vi "Get Tables.vi"(8 "error in (no error)":errorcluster, 11 "xwpfDocument in":refnum<class "xwpfDocument.lvclass">) -> (0 "error out":errorcluster, 2 "Tables":refnum<class "xwpfTable.lvclass">[](array[class]), 3 "xwpfDocument out":refnum<class "xwpfDocument.lvclass">)   [LabVIEW 2017, in "Word_Specific.lvlib" / "xwpfDocument.lvclass"]
uses:
  xwpfDocument.lvclass
  xwpfTable/xwpfTable.lvclass
  xwpfDocument.lvclass/xwpfDocument.ctl
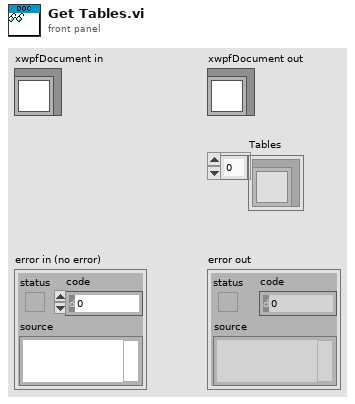
[diagram p1: front panel]
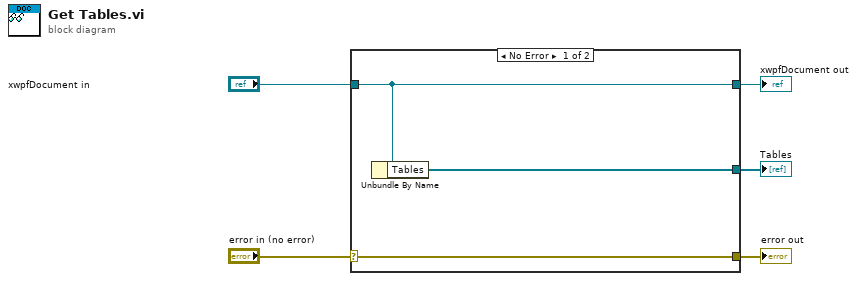
[diagram p0: block diagram]
diagram:
  n1 = case shown="No Error" "error in (no error)" {
    selector: "error in (no error)" -> [w8 w9]
    tunnel: [w8 w9] -> w4
    tunnel: [w7 w10] -> w2
    tunnel: "xwpfDocument in" -> [w7 w10]
    tunnel: [w6 _] -> w1
    frame No Error {
      n2 = Unbundle By Name(w7) -> ("Tables"=w6:refnum<class "xwpfTable.lvclass">[])
    }
    frame Error {
    }
  }
  "error out" <- w4
  "xwpfDocument out" <- w2
  "Tables" <- w1
